vi "Event Timing Measure 1.1 In Place Output Read Structure.vi"(7 "Device outputs in":dbl[](array[numeric]), 8 "error in (no error)":errorcluster, 9 "FPGA ref in":T1, 11 "1.1 Event Timing Measure in":T2) -> (0 "error out":errorcluster, 1 "FPGA ref out":T1, 3 "1.1 Event Timing Measure out":T2, 5 "Device outputs out":dbl[](array[numeric]))   [LabVIEW 2020, in "Engine Simulation Toolkit Engine.lvlib"]
uses:
  Engine Simulation Toolkit Engine.lvlib
  Shared/1.1 Event Timing Measure Engine Data.ctl
  Shared/1.0 Event Timing Measure FIFO Idxs.ctl
  Event Timing Measure 1.0 Output Ref.ctl
  <vilib>/Utility/error.llb/Error Cluster From Error Code.vi
  <vilib>/rvi/errors/niLvFpgaAdjustHostInterfaceError.vi
  <vilib>/rvi/interface/nirviReadWriteControl/nirviReadWriteControl.xnode
  NiFpgaLv.dll
  <vilib>/rvi/interface/Simulation/niFpgaSimulationCallBeginRW.vi
  Shared/Engine Simulation Toolkit Shared.lvlib
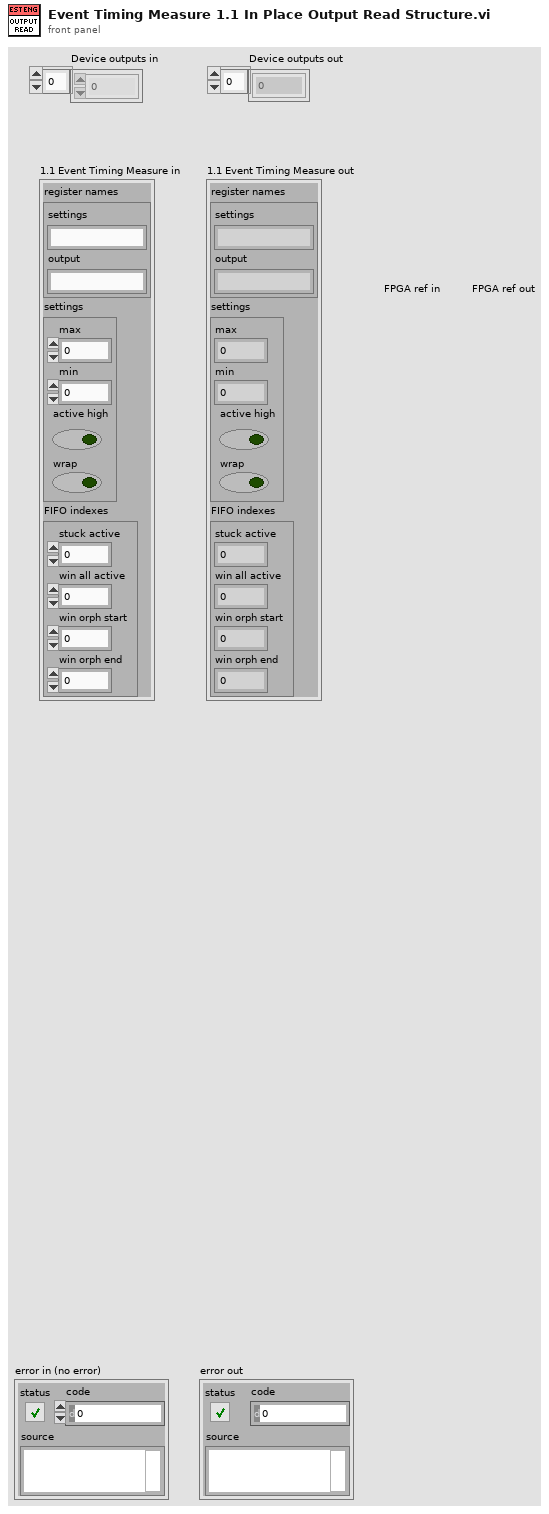
[diagram p1: front panel]
types:
  T1 = typedef "Engine Simulation Toolkit Engine.lvlib/Event Timing Measure 1.0 Output Ref.ctl" = refnum<k20>
  T2 = typedef "Engine Simulation Toolkit Shared.lvlib/1.1 Event Timing Measure Engine Data.ctl" = cluster{"register names":cluster{"settings":string, "output":string}, "settings":cluster{"max":u16, "min":u16, "active high":bool, "wrap":bool}, "FIFO indexes":T3}
  T3 = typedef "Engine Simulation Toolkit Shared.lvlib/1.0 Event Timing Measure FIFO Idxs.ctl" = cluster{"stuck active":i32, "win all active":i32, "win orph start":i32, "win orph end":i32}
  T4 = cluster{"stuck active":bool, "window all active":bool, "window orphan start":bool, "window orphan end":bool}
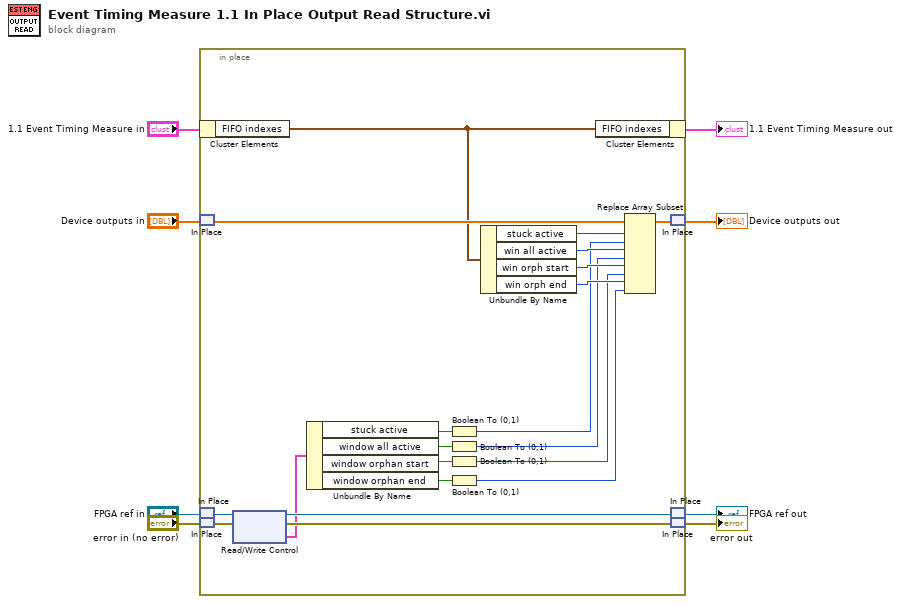
[diagram p0: block diagram]
diagram:
  n1 = in-place {
    n2 = in-place-cluster #1("1.1 Event Timing Measure in") -> ("FIFO indexes"=w21:T3)
    n3 = in-place-match #2("Device outputs in") -> (w23:dbl[])
    n4 = in-place-match #3("FPGA ref in") -> (w27:T1)
    n5 = in-place-match #4("error in (no error)") -> (w28:errorcluster)
    n6 = xnode "Read/Write Control"("FPGA VI Reference In"=w27, "error in"=w28) -> ("FPGA VI Reference Out"=w26:T1, "error out"=w25:errorcluster, "Value"=w24:T4)
    n7 = Unbundle By Name(w24) -> ("stuck active"=w16:bool, "window all active"=w15:bool, "window orphan start"=w14:bool, "window orphan end"=w13:bool)
    n8 = Boolean To (0,1)(Boolean=w16) -> (0, 1=w12:i16)
    n9 = Boolean To (0,1)(Boolean=w15) -> (0, 1=w11:i16)
    n10 = Boolean To (0,1)(Boolean=w14) -> (0, 1=w10:i16)
    n11 = Boolean To (0,1)(Boolean=w13) -> (0, 1=w9:i16)
    n12 = Unbundle By Name(w21) -> ("stuck active"=w20:i32, "win all active"=w19:i32, "win orph start"=w18:i32, "win orph end"=w17:i32)
    n13 = in-place-cluster #1("FIFO indexes"=w21) -> (→"1.1 Event Timing Measure out":T2)
    n14 = Replace Array Subset(array=w23, new element #1=w12, index #1=w20, new element #2=w11, index #2=w19, new element #3=w10, index #3=w18, new element #4=w9, index #4=w17) -> (w22:dbl[])
    n15 = in-place-match #2(w22) -> (→"Device outputs out":dbl[])
    n16 = in-place-match #3(w26) -> (→"FPGA ref out":T1)
    n17 = in-place-match #4(w25) -> (→"error out":errorcluster)
  }
